vi "RSZVB Set Output Port Bits.vi"(8 "error in (no error)":errorcluster {"code" format="%.0x"}, 9 "Port Bits (0)":i32, 10 "Output Port (A)":i32(ring) items=["A", "B"], 11 "VISA session":refnum<visa-resource-name>) -> (0 "error out":errorcluster {"code" format="%.0x"}, 3 "dup VISA session":refnum<visa-resource-name>)   [LabVIEW 2011]
doc: "This VI sets a channel-dependent bit pattern to the output ports A or B of the Universal Interface (option R&S ZVAB-B14). The channel bits are combined with the (static) output bits defined via CONTrol:HANDler:A|B[:DATA] using a logical \"or\" operation. The channel bits must be defined while the channel is active (CONTrol:NSELect <Ch>); the corresponding signals will be in effect while the channel is measured (dynamic output signals).\n\nRemote-control command(s):\nCONTrol:AUXiliary:A[:DATA]\nCONTrol:AUXiliary:B[:DATA]"
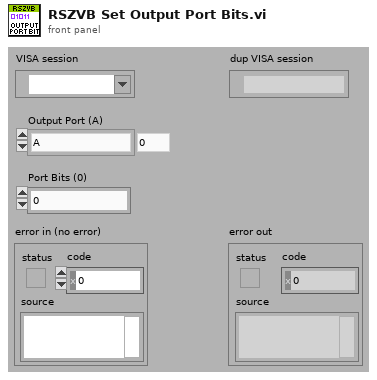
[diagram p1: front panel]
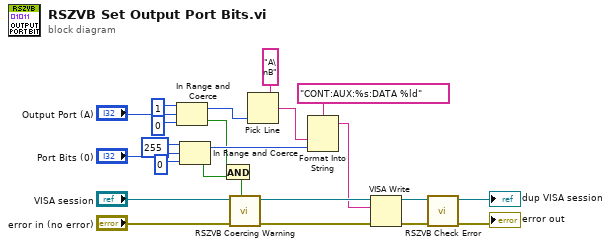
[diagram p0: block diagram]
diagram:
  n1 = In Range and Coerce(upper limit=1, x="Output Port (A)", lower limit=0) -> (coerced(x)=w4:i32, In Range?=w3:bool)
  n2 = In Range and Coerce(upper limit=255, x="Port Bits (0)", lower limit=0) -> (coerced(x)=w5:i32, In Range?=w2:bool)
  n3 = And(x=w3, y=w2) -> (x .and. y?=w1:bool)
  n4 = call "RSZVB Coercing Warning.vi"("In Range?"=w1, "error in (no error)"="error in (no error)", "VISA session"="VISA session") -> ("error out"=w19:errorcluster, "dup VISA session"=w20:refnum<visa-resource-name>)  [unwired: 7 in]
  n5 = Pick Line(multi-line string="A\nB", line index=w4) -> (output string=w6:string)  [unwired: 1 in]
  n6 = Format Into String(format string="CONT:AUX:%s:DATA %ld", w6, w5) -> (resulting string=w16:string)  [unwired: 2 in, 1 out]
  n7 = VISA Write(VISA resource name=w20, write buffer=w16, error in (no error)=w19) -> (VISA resource name out=w17:refnum<visa-resource-name>, error out=w18:errorcluster)  [unwired: 1 out]
  n8 = call "RSZVB Check Error.vi"("error in (no error)"=w18, "VISA session"=w17) -> ("error out"=→"error out":errorcluster, "dup VISA session"=→"dup VISA session":refnum<visa-resource-name>)  [unwired: 8 in]
